vi "lab_4_group_10_main.vi"() -> ()   [LabVIEW 2020]
panel:
  out "Waveform Chart":dbl(graph)
  in  "U(Manual)\nm3/sec":dbl
  out "Manual 2":bool
  out "PID ON":bool
  in  "PID on/off":bool
  in  "H2,ref\n[m]":dbl
  in  "Kd":dbl
  in  "Ki":dbl
  in  "Kp":dbl
  out "U (PID)\n[m³/s]":dbl
  in  "hss,2\n[m]":dbl
  out "KmVs (steady-\nstate-inflow)\n[m³/s]":dbl
  out "hss,1\n[m]":dbl
  out "H2 (H2 = h2 -hss,2)\n[m]":dbl(graph)
  out "H1 (H1 = h1 - hss,1)\n[m]":dbl(graph)=100.0
  out "Slide 4":u8(slide) scale=0.0..100.0
  out "Tank 2 is empty":bool
  out "Tank 2 is full":bool
  out "Tank 2":dbl(slide) scale=0.0..100.0
  out "Slide 1":u8(slide) scale=0.0..100.0
  out "Slide 3":u8(slide) scale=0.0..100.0
  out "Slide 2":u8(slide) scale=0.0..100.0
  out "Tank 1 is full":bool
  out "Tank 1 is empty":bool
  in  "?":bool
  out "Tank 1":dbl(slide) scale=0.0..100.0
  # "h1\n[m]"
  # "h2\n[m]"
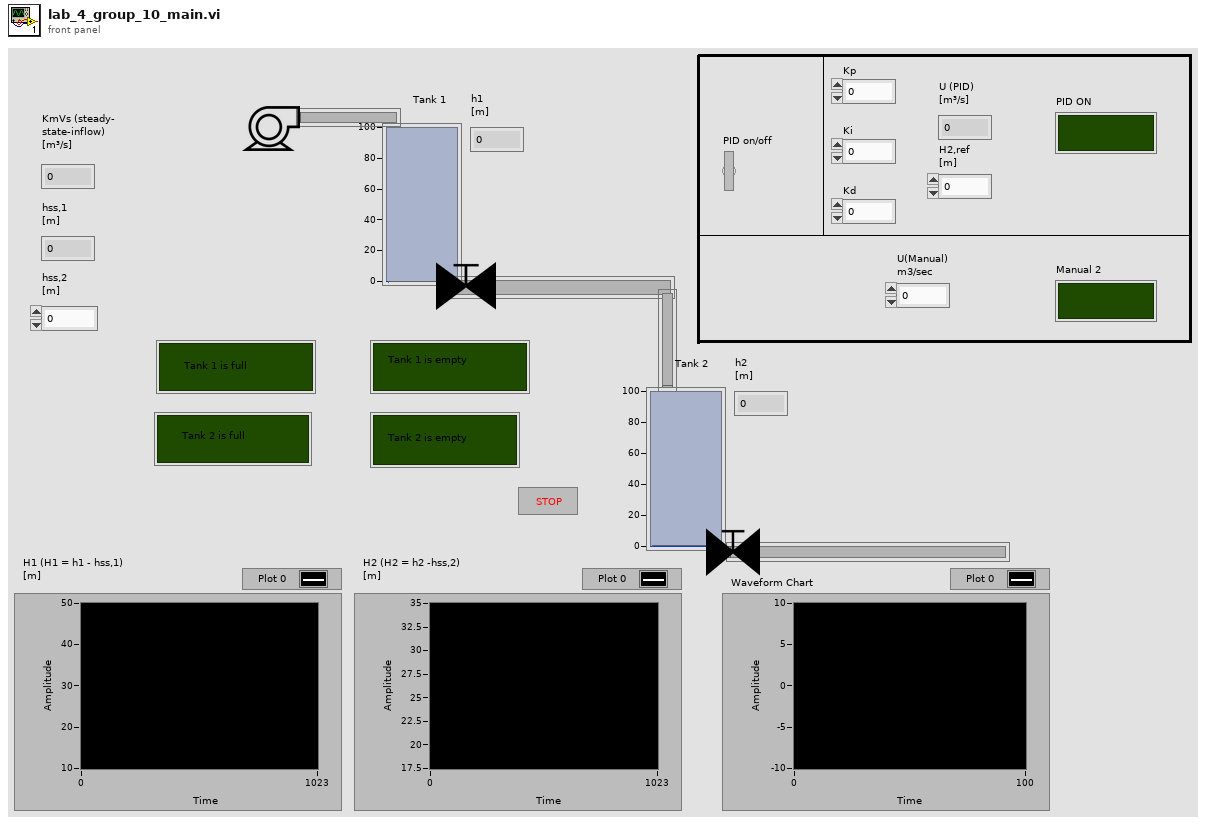
[diagram p1: front panel]
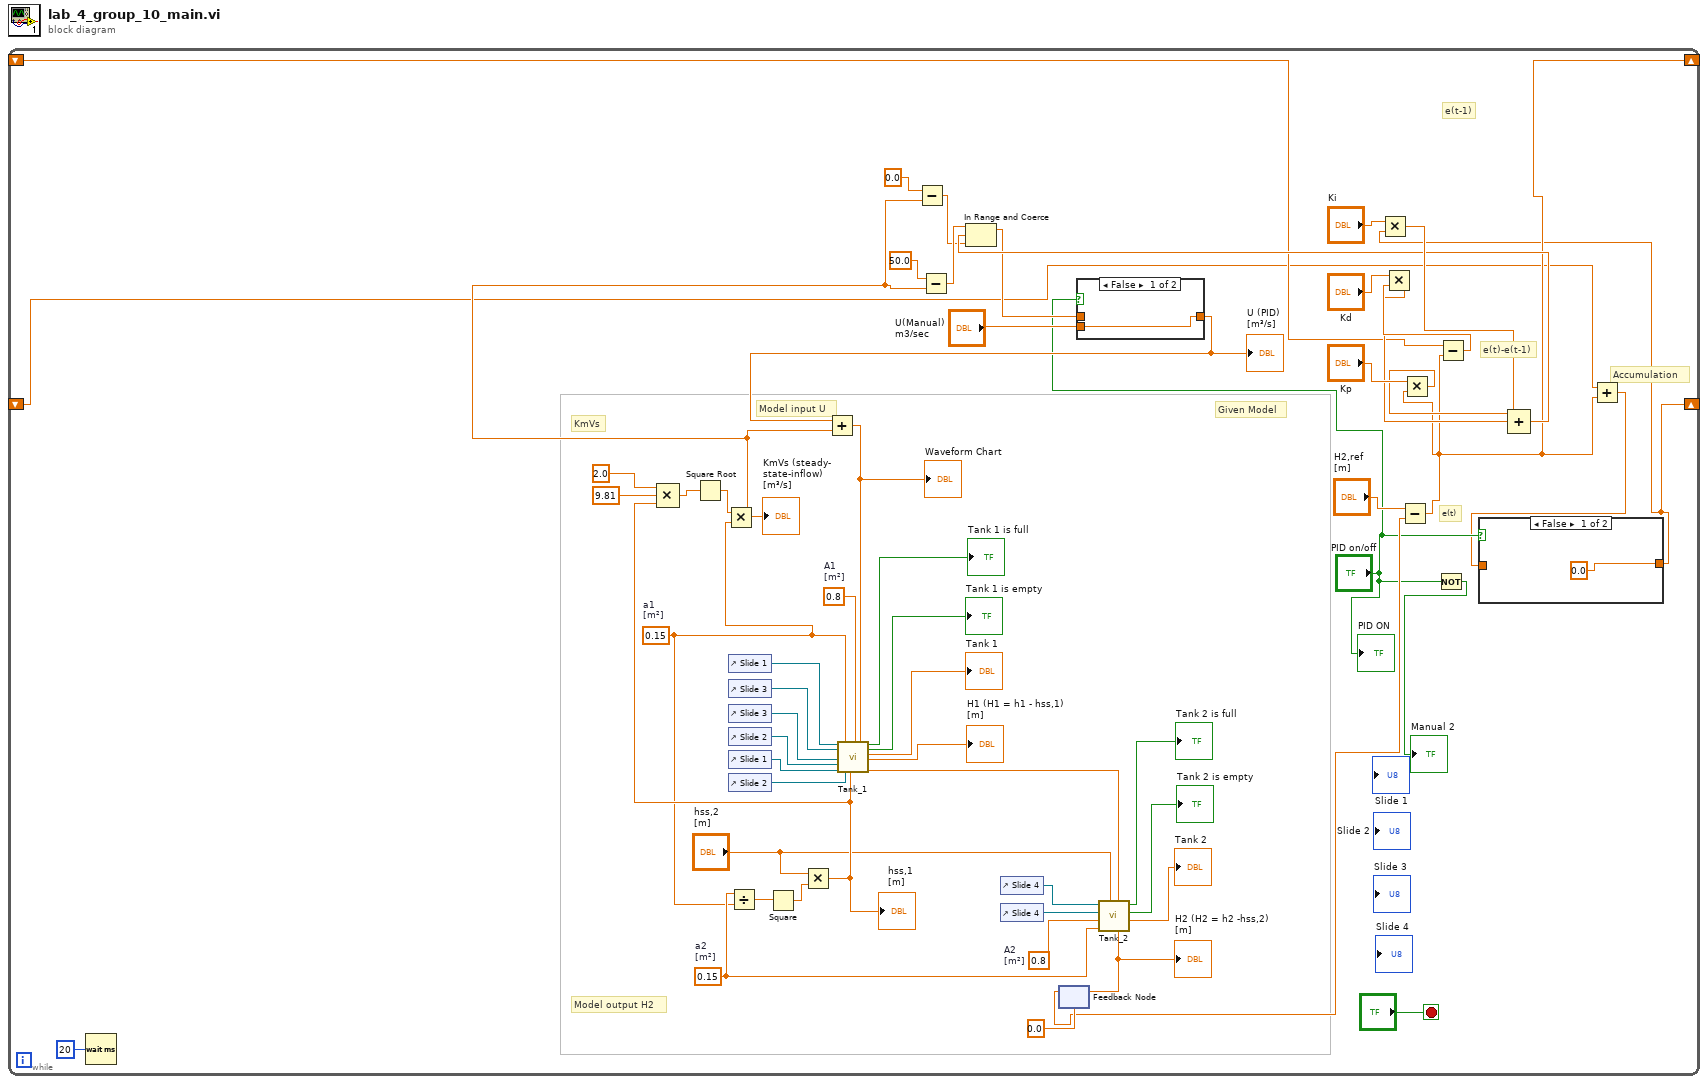
[diagram p0: block diagram]
diagram:
  n1 = while {
    shift-right: [w7] -> _
    shift-left: _ -> [w9]
    shift-right: [w4] -> _
    shift-left: _ -> [w6]
    stop <- "?" stop-if-true
    w44 = 0.15  # a2 [m²]
    w54 = 0.8  # A2 [m²]
    w29 = 0.15  # a1 [m²]
    w37 = 0.8  # A1 [m²]
    # "Accumulation"
    # "e(t-1)"
    # "e(t)-e(t-1)"
    # "e(t)"
    # "KmVs"
    # "Model output H2"
    # "Model input U"
    # "Given Model"
    n2 = Wait (ms)(milliseconds to wait=u32 20 ("millisecond timer value")) -> ()  [unwired: 1 out]
    n3 = control-ref of="Slide 1"() -> (w51:refnum<vi>)
    n4 = control-ref of="Slide 3"() -> (w50:refnum<vi>)
    n5 = control-ref of="Slide 3"() -> (w49:refnum<vi>)
    n6 = control-ref of="Slide 2"() -> (w48:refnum<vi>)
    n7 = control-ref of="Slide 1"() -> (w47:refnum<vi>)
    n8 = control-ref of="Slide 2"() -> (w46:refnum<vi>)
    n9 = Divide(x=w44, y=w29) -> (x/y=w53:dbl)
    n10 = Square(x=w53) -> (x^2=w52:dbl)
    n11 = Multiply(x="hss,2\n[m]", y=w52) -> (x*y=w41:dbl)
    "hss,1\n[m]" <- w41
    n12 = Compound Arithmetic op=MULTIPLY(2.0, 9.81, w41) -> (w40:dbl)
    n13 = Square Root(x=w40) -> (sqrt(x)=w39:dbl)
    n14 = Multiply(x=w39, y=w29) -> (x*y=w16:dbl)
    "KmVs (steady-\nstate-inflow)\n[m³/s]" <- w16
    n15 = Subtract(x=0.0 ("y"), y=w16) -> (x-y=w2:dbl)
    n16 = Subtract(x=50.0, y=w16) -> (x-y=w3:dbl)
    n17 = control-ref of="Slide 4"() -> (w57:refnum<vi>)
    n18 = control-ref of="Slide 4"() -> (w56:refnum<vi>)
    n19 = feedback #1(0.0) -> (w25:dbl)
    n20 = Subtract(x="H2,ref\n[m]", y=w25) -> (x-y=w7:dbl)
    n21 = Multiply(x="Kp", y=w7) -> (x*y=w23:dbl)
    n22 = Not(x="PID on/off") -> (.not. x?=→"Manual 2":bool)
    n23 = Subtract(x=w9, y=w7) -> (x-y=w20:dbl)
    n24 = Multiply(x="Kd", y=w20) -> (x*y=w19:dbl)
    n25 = Add(x=w6, y=w7) -> (x+y=w5:dbl)
    n26 = case shown="False" "PID on/off" {
      tunnel: w5 -> [_ w60]
      tunnel: [0.0 ("x") w60] -> w4
      frame False {
      }
      frame True {
      }
    }
    n27 = Multiply(x="Ki", y=w4) -> (x*y=w18:dbl)
    n28 = Compound Arithmetic op=ADD(w23, w19, w18) -> (w13:dbl)
    n29 = In Range and Coerce(upper limit=w3, x=w13, lower limit=w2) -> (coerced(x)=w12:dbl)  [unwired: 1 out]
    n30 = case shown="False" "PID on/off" {
      tunnel: w12 -> [_ w62]
      tunnel: [w61 w62] -> w11
      tunnel: "U(Manual)\nm3/sec" -> [w61 _]
      frame False {
      }
      frame True {
      }
    }
    "U (PID)\n[m³/s]" <- w11
    n31 = Add(x=w11, y=w16) -> (x+y=w1:dbl)
    "Waveform Chart" <- w1
    n32 = call "Tank_1.vi"("Slide in"=w51, "Slide 3"=w50, "Slide Refnum"=w49, "Slide Refnum 2"=w48, "Slide Refnum 3"=w47, "a1 (Crosssection of connecting valve)\n[m²]"=w29, "Slide 2"=w46, "hss,1\n[m]"=w41, "A1 (Crosssection of Tank 1)\n[m²"=w37, "KmVi\n[m³/s]"=w1) -> ("Tank 1 is full"=→"Tank 1 is full":bool, "Tank 1 is empty"=→"Tank 1 is empty":bool, "h1\n[m]"=→"Tank 1":dbl, "H1\n[m]"=→"H1 (H1 = h1 - hss,1)\n[m]":dbl, "outflow\n[m³/s]"=w35:dbl)  [unwired: 5 in]
    n33 = call "Tank_2.vi"("Inflow\n[m³/s]"=w35, "hss,2\n[m]"="hss,2\n[m]", "a2 (outlet of Tank 2)\n[m²]"=w44, "A2 (Crosssection of Tank 2)\n[m²] 2"=w54, "Slide 4"=w56, "Slide in"=w57) -> ("h2\n[m]"=→"Tank 2":dbl, "Tank 2 is empty"=→"Tank 2 is empty":bool, "Tank 2 is full"=→"Tank 2 is full":bool, "H2\n[m]"=w32:dbl)  [unwired: 2 in]
    "H2 (H2 = h2 -hss,2)\n[m]" <- w32
    n34 = feedback-in #1(w32) -> ()
    "PID ON" <- "PID on/off"
  }
